vi "Clear Context.vi"(8 "error in (no error)":errorcluster, 11 "Process In":refnum<class "Debug View.lvclass">) -> (0 "error out":errorcluster, 3 "Process Out":refnum<class "Debug View.lvclass">)   [LabVIEW 2020]
doc: "Framework method for clearing the context of a process."
uses:
  Debug View.lvclass
  Debug View.lvclass/Debug View.ctl
  <vilib>/Utility/error.llb/Clear Errors.vi
  <vilib>/Utility/error.llb/Error Cluster From Error Code.vi
  <vilib>/ErrorRing/Error Ring.xnode
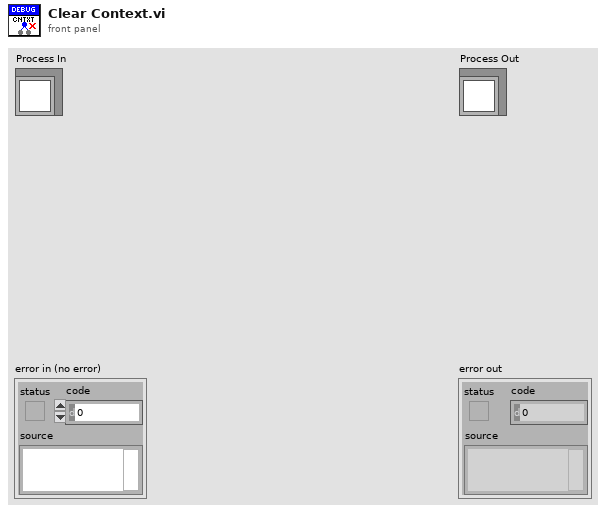
[diagram p1: front panel]
types:
  T1 = typedef "Lifecycle State.ctl" = enum16{"Uninitialized", "Initialized", "Started", "Running", "Stopped", "Finished"}
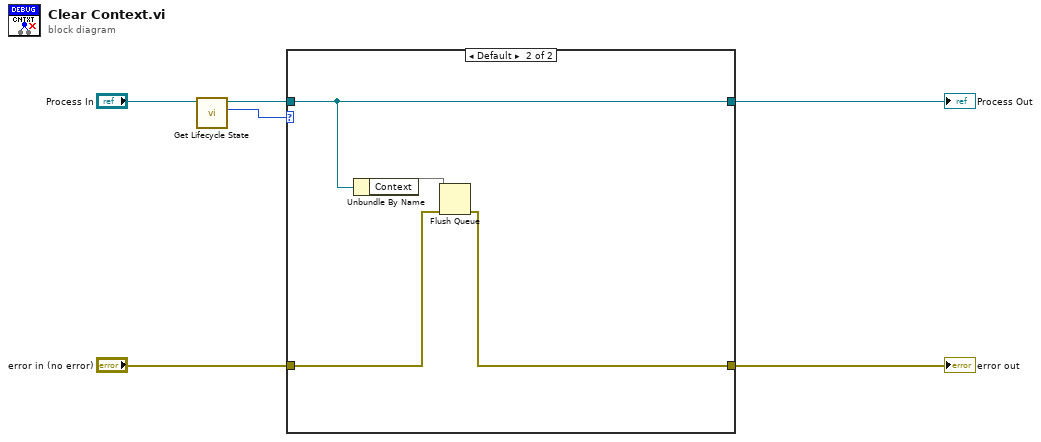
[diagram p0: block diagram]
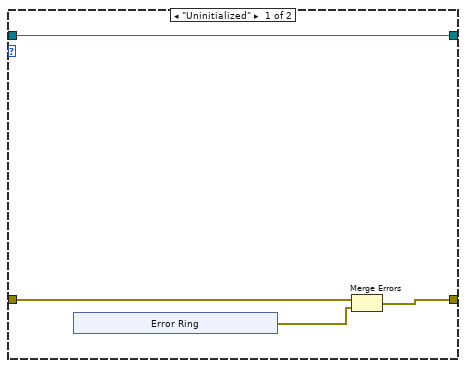
[diagram p2: hidden frame]
diagram:
  n1 = call "Get Lifecycle State.vi"("Process In"="Process In") -> ("Lifecycle State"=w2:T1, "Process Out"=w3:refnum<class "Debug View.lvclass">)  [unwired: 7 in, 2 out]
  n2 = case shown="Default" w2 {
    tunnel: [w10 w18] -> w6
    tunnel: [w8 w16] -> w5
    tunnel: w3 -> [w10 w18]
    tunnel: "error in (no error)" -> [w9 w15]
    frame "Uninitialized" {
      n3 = xnode "Error Ring"() -> ("error out"=w7:errorcluster)
      n4 = Merge Errors(w9, w7) -> (w8:errorcluster)
    }
    frame Default {
      n5 = Unbundle By Name(w18) -> ("Context"=w17)
      n6 = Flush Queue(queue=w17, error in (no error)=w15) -> (error out=w16:errorcluster)  [unwired: 2 out]
    }
  }
  "error out" <- w5
  "Process Out" <- w6
